vi "FINamedPosition.vi"(2 "Position":string, 3 "FI":string, 9 "error in (no error)":errorcluster) -> (0 "X":i32, 1 "Y":i32, 5 "Z":i32, 6 "error out":errorcluster)   [LabVIEW 2009]
uses:
  Controls/FIManagerData.ctl
  Controls/FINamedPosition.ctl
  <vilib>/Utility/config.llb/NI_LVConfig.lvlib
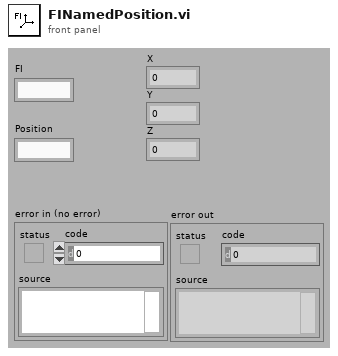
[diagram p1: front panel]
types:
  T1 = typedef "FIManagerData.ctl" = cluster{"ReferencePosition":T2, "OffsetsPositions":T2[]}
  T2 = typedef "FINamedPosition.ctl" = cluster{"Name":string, "X":i32, "Y":i32, "Z":i32}
  T3 = typedef "NI_LVConfig.lvlib/Config Data RefNum.ctl" = refnum<k1>
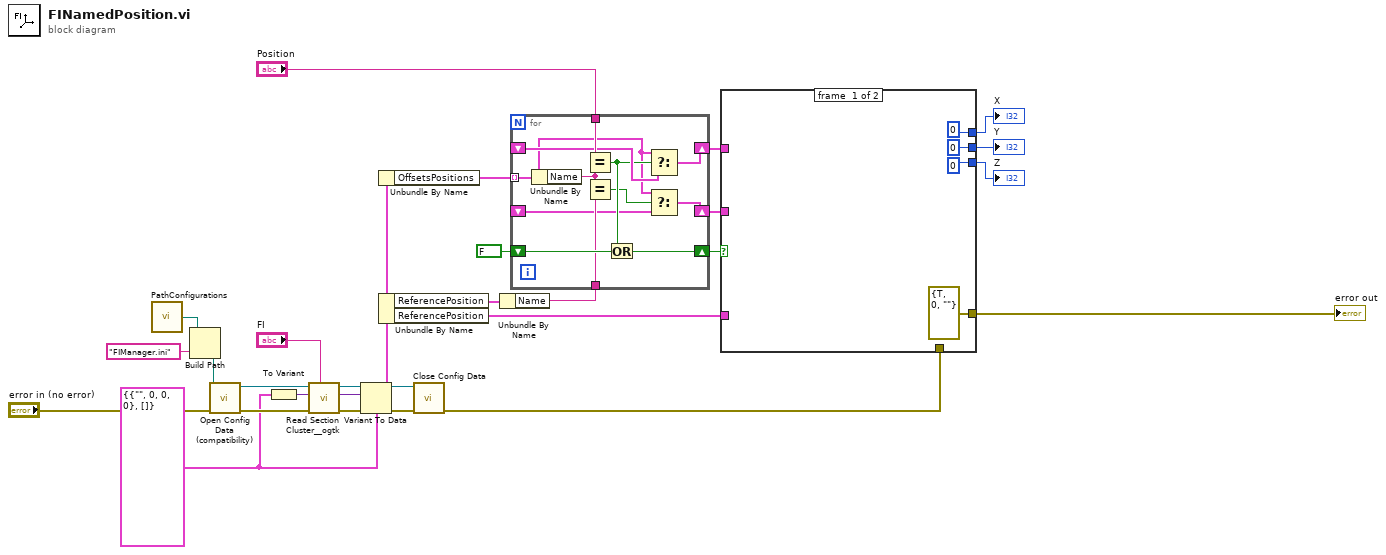
[diagram p0: block diagram]
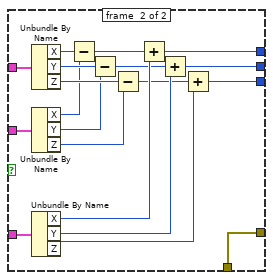
[diagram p2: hidden frame]
diagram:
  w18 = T1 {"ReferencePosition"={"Name"="", "X"=0, "Y"=0, "Z"=0}, "OffsetsPositions"=[]} ("FIManagerData")
  n1 = call "PathConfigurations.vi"() -> ("OhanaOS Path"=w28:path)
  n2 = Build Path(base path=w28, name or relative path="FIManager.ini") -> (appended path=w26:path)
  n3 = call <vilib>:"Open Config Data (compatibility).vi"("error in (no error)"="error in (no error)", "configuration file path"=w26) -> ("error out"=w25:errorcluster, "refnum"=w24:T3)  [unwired: 7 in, 1 out]
  n4 = To Variant(anything=w18) -> (Variant=w22:variant)
  n5 = call <userlib>:"Read Section Cluster__ogtk.vi"("section (optional)"="FI", "error in (no error)"=w25, "Section Formatted Cluster Type"=w22, "refnum"=w24) -> ("error out"=w21:errorcluster, "Section Formatted Cluster"=w19:variant, "dup refnum"=w23:T3)  [unwired: 5 out]
  n6 = Variant To Data(error in=w21, Variant=w19, type=w18) -> (error out=w20:errorcluster, data=w14:T1)
  n7 = Unbundle By Name(w14) -> ("OffsetsPositions"=w17:T2[])
  n8 = Unbundle By Name(w14) -> ("ReferencePosition"=w11:T2, "ReferencePosition"=w12:T2)
  n9 = call <vilib>:"Close Config Data.vi"("error in (no error)"=w20, "refnum"=w23) -> ("error out"=w5:errorcluster)  [unwired: 1 in, 8 out]
  n10 = Unbundle By Name(w11) -> ("Name"=w10:string)
  n11 = for {
    tunnel: w17 -> [w32] mode=indexing
    tunnel: "Position" -> [w40]
    shift-right: [w33] -> w13
    shift-left: _ -> [w39]
    shift-right: [w38] -> w8
    shift-left: FALSE -> [w37]
    tunnel: w10 -> [w34]
    shift-right: [w31] -> w9
    shift-left: _ -> [w29]
    n12 = Unbundle By Name(w32) -> ("Name"=w35:string)
    n13 = Equal?(x=w40, y=w35) -> (x = y?=w36:bool)
    n14 = Equal?(x=w35, y=w34) -> (x = y?=w30:bool)
    n15 = Or(x=w36, y=w37) -> (x .or. y?=w38:bool)
    n16 = Select(t=w32, s=w36, f=w39) -> (s? t:f=w33:T2)
    n17 = Select(t=w32, s=w30, f=w29) -> (s? t:f=w31:T2)
  }
  n18 = case shown="False" w8 {
    tunnel: w13 -> [_ w63]
    tunnel: w12 -> [_ w62]
    tunnel: w9 -> [_ w58]
    tunnel: w5 -> [_ w48]
    tunnel: [errorcluster {"status"=TRUE, "code"=0, "source"=""} ("error out") w48] -> w4
    tunnel: [0 w47] -> w3
    tunnel: [0 w46] -> w2
    tunnel: [0 w45] -> w1
    frame #0 {
    }
    frame #1 {
      n19 = Unbundle By Name(w63) -> ("X"=w61:i32, "Y"=w60:i32, "Z"=w59:i32)
      n20 = Unbundle By Name(w58) -> ("X"=w57:i32, "Y"=w56:i32, "Z"=w55:i32)
      n21 = Unbundle By Name(w62) -> ("X"=w54:i32, "Y"=w53:i32, "Z"=w52:i32)
      n22 = Subtract(x=w61, y=w57) -> (x-y=w51:i32)
      n23 = Subtract(x=w60, y=w56) -> (x-y=w50:i32)
      n24 = Subtract(x=w59, y=w55) -> (x-y=w49:i32)
      n25 = Add(x=w51, y=w54) -> (x+y=w47:i32)
      n26 = Add(x=w50, y=w53) -> (x+y=w46:i32)
      n27 = Add(x=w49, y=w52) -> (x+y=w45:i32)
    }
  }
  "error out" <- w4
  "X" <- w3
  "Y" <- w2
  "Z" <- w1
